vi "REF_X_COM8_hex_VE_FP_STOP_BR_slew_LIM2_Si3540.vi"() -> ()   [LabVIEW 2009]
uses:
  <vilib>/Instr/_visa.llb/VISA Configure Serial Port (Instr).vi
panel:
  out "slew velocity mm/sec":dbl
  out "slew length mm":dbl
  in  "Slew Cancel":bool
  out "Position mm":dbl
  out "offset":dbl
  out "mm/rev":dbl
  out "step/rev":u32
  out "rev/sec":dbl
  in  "Slew Length":i32 min=-99000 max=101000 step=100
  out "Slew Ready":bool
  in  "Slew Set":bool
  in  "Slew Go":bool
  in  "Velocity":dbl
  in  "Slew Velocity":dbl=0.0043 min=0.0042 max=0.105 step=0.0042
  in  "Backlash":i32
  in  "Stop":bool
  out "In Range?":bool
  out "Current Values":i32 max=2000
  out "Status":string
  in  "Go":bool
  in  "Move to":i32=-20000 min=-100000 max=100000 step=500
  out "MINPOS":i32=-94296
  out "MAXPOS":i32=-34296
  out "COM PORT":refnum<visa-resource-name>="COM5"
  # "REF Y"
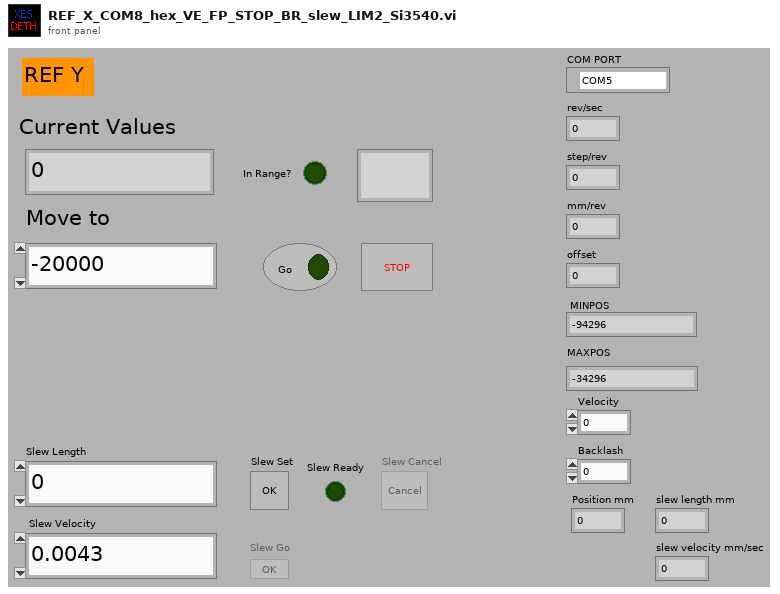
[diagram p1: front panel]
types:
  T1 = enum8{"Enabled", "Disabled", "Disabled and Grayed Out"}
  T2 = enum16{"Power-up Signature", "Accel Rate", "Accel Max", "Bit Rate", "Buffer Status", "Change Current", "Commence Jogging", "Change Jog Speed", "Continue", "Define Address", "Distance for FC,FM,FO,FY", "Decel Rate", "Distance or Position", "Define Limits", "Encoder Deadband", "Encoder Function", "Encoder Position", "Encoder Ratio", "Feed to Length with Speed Change", "Feed to Length", "Feed to Sensor with Mask Dist", "Feed to Length & Set Output", "Feed to Position", "Feed to Sensor", "Feed to Sensor w/safety", "Follow Handwheel", "Immediate Distance?", "Immediate Encoder?", "Immediate Low Output", "Immediate High Output", "Immediate Position?", "Input Status?", "Jog Accel/Decel", "Jog Disable", "Jog Enable", "Jog Speed", "Motor Disable", "Motor Enable", "Microstep Resolution", "Power up Current", "Power up Mode", "Pause", "Request Status", "Revision Level?", "Seek Home", "Stop Jogging", "Stop & Kill Buffer", "Set Output", "Set ABS Position", "Send String", "Stop", "Velocity for Speed Change", "Velocity Setting", "Wait for Input", "Wait Time"}
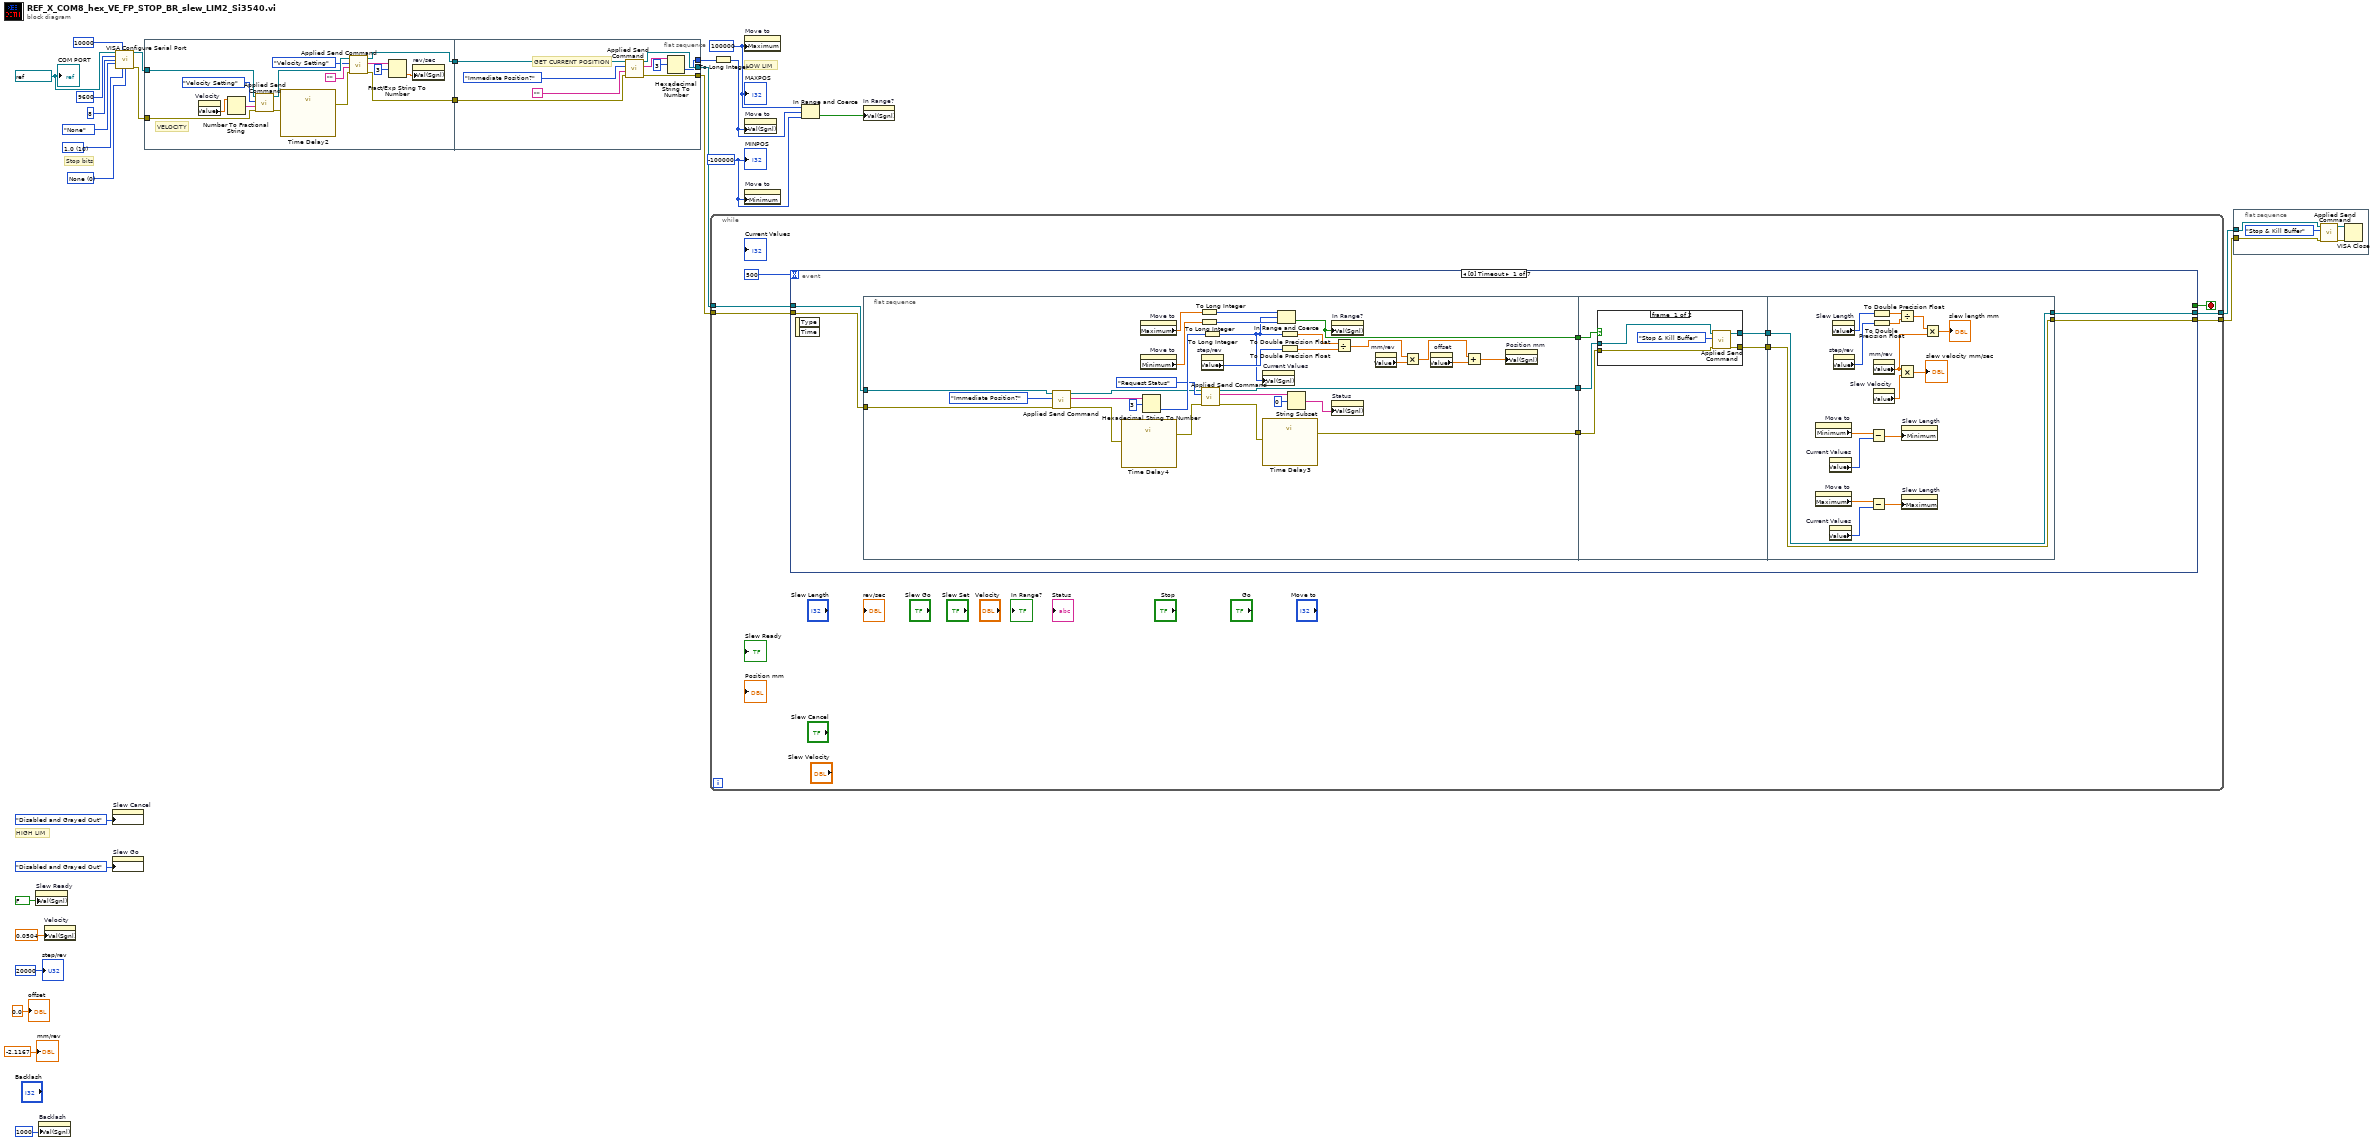
[diagram p0: block diagram]
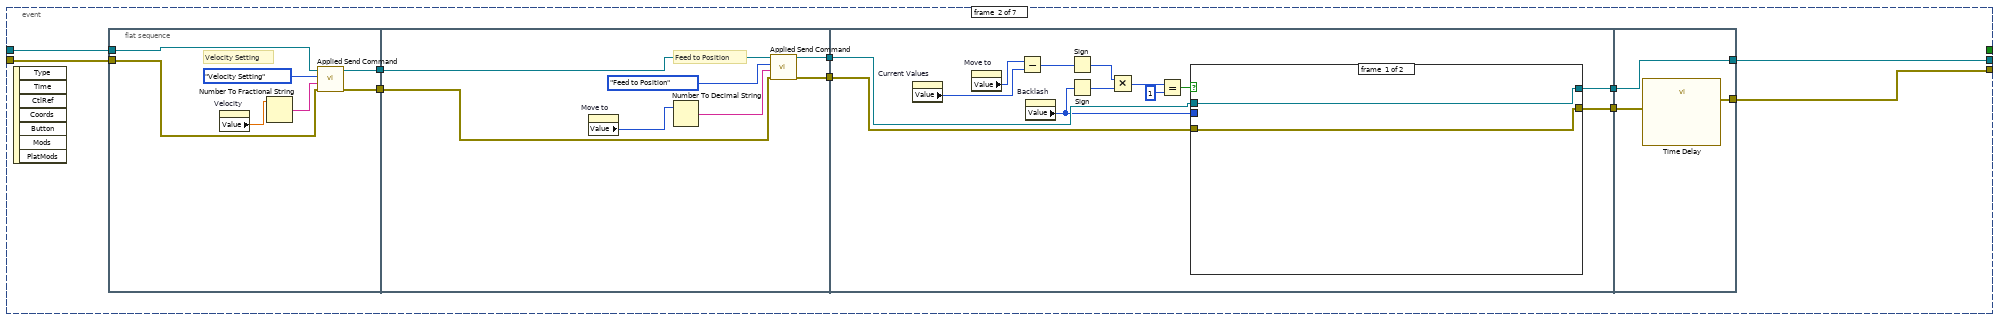
[diagram p3: hidden frame]
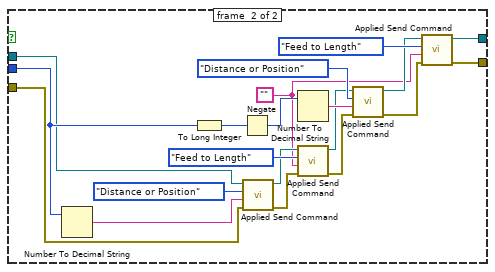
[diagram p4: hidden frame]
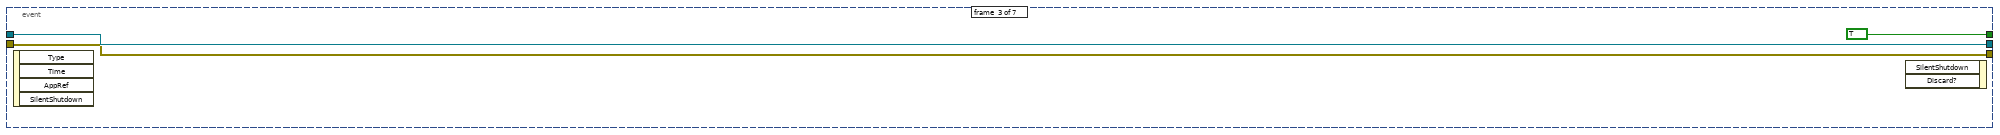
[diagram p5: hidden frame]
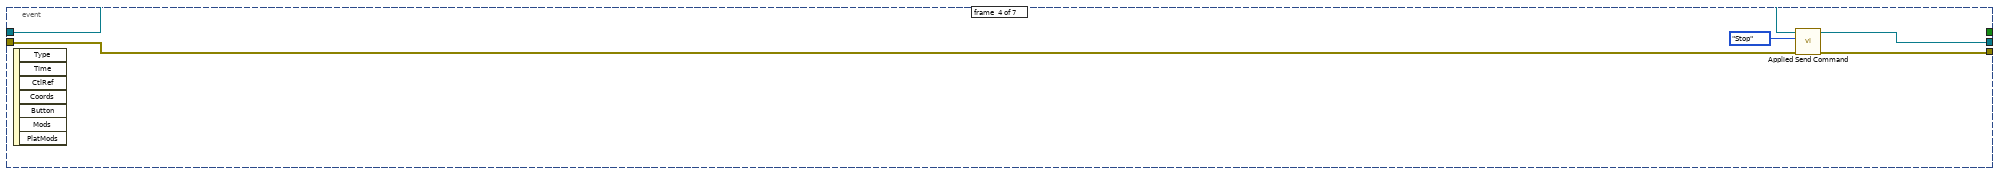
[diagram p6: hidden frame]
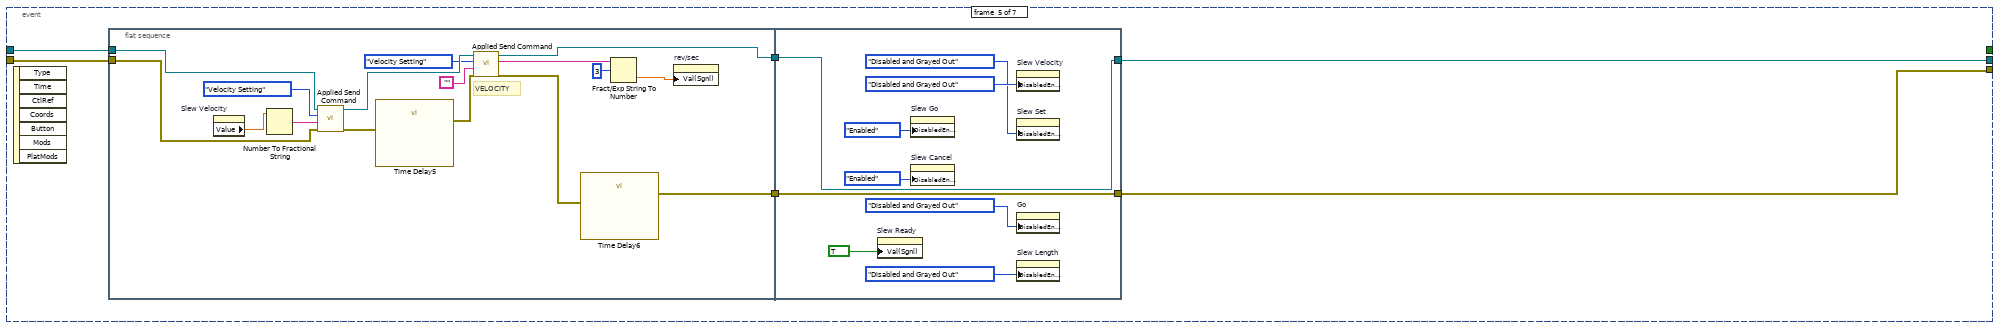
[diagram p7: hidden frame]
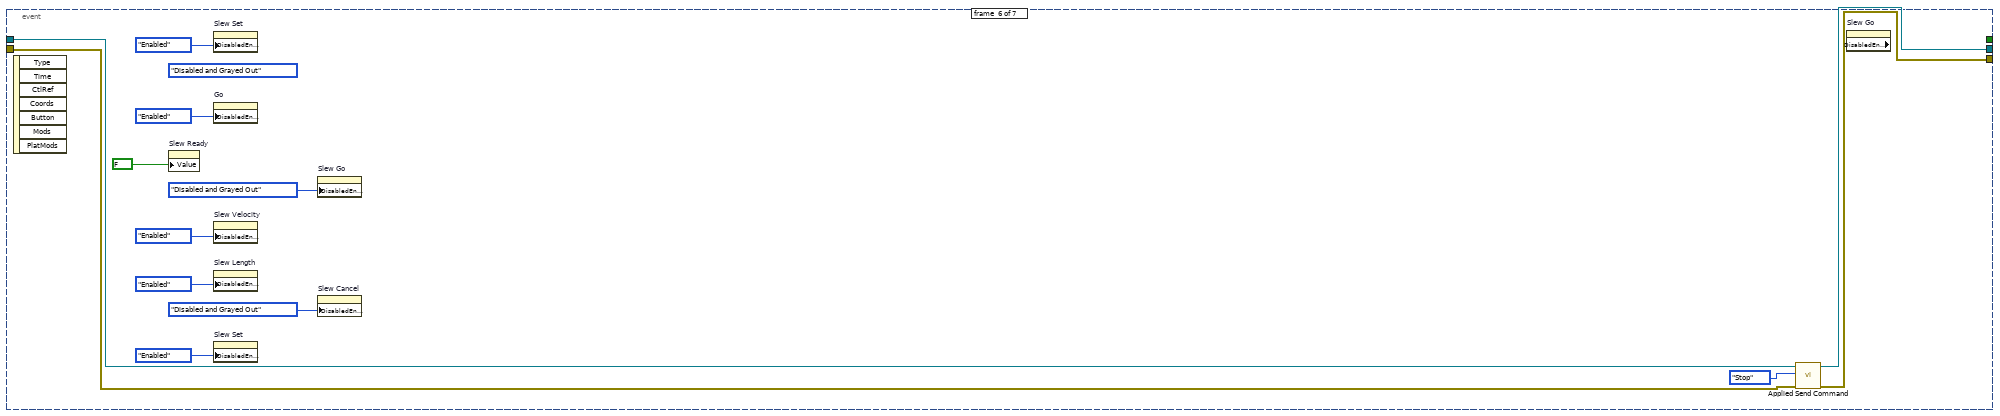
[diagram p8: hidden frame]
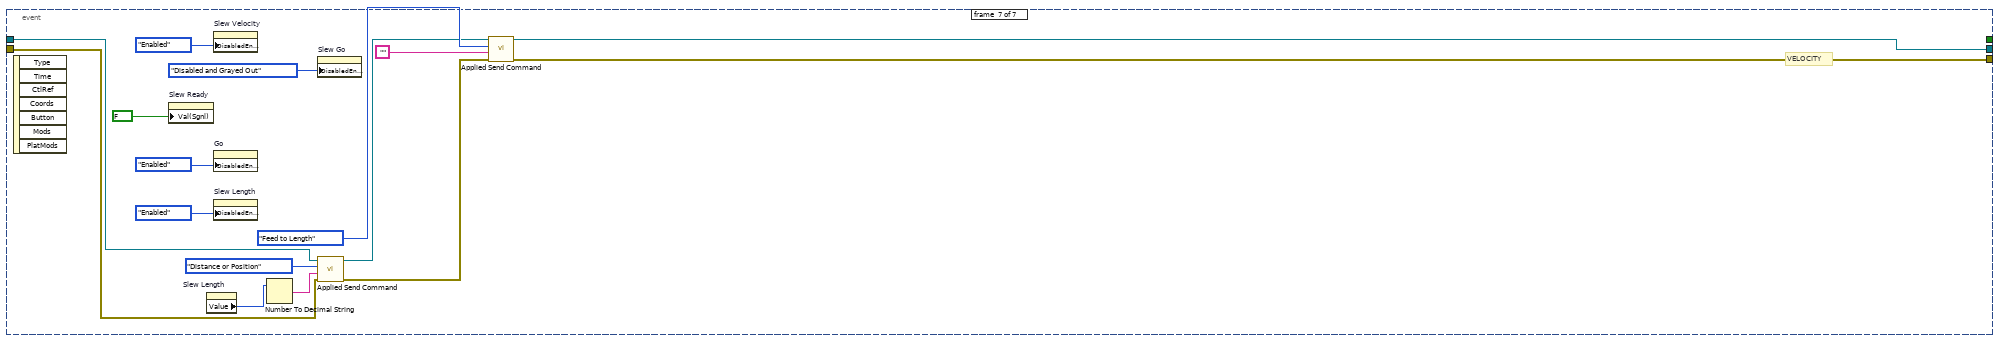
[diagram p9: hidden frame]
diagram:
  w14 = -100000 ("lower limit")
  w13 = 100000 ("upper limit")
  w22 = refnum<visa-resource-name> "COM8" ("COM PORT")
  w24 = u16 0 items=["None", "XON/XOFF", "RTS/CTS", "XON/XOFF & RTS/CTS", "DTR/DSR", "XON/XOFF & DTR/DSR"] ("flow control (0:none)")
  w25 = u16 10 items=["1.0"=10, "1.5"=15, "2.0"=20] ("stop bits (10: 1 bit)")
  # "HIGH LIM"
  # "LOW LIM"
  # "Stop bits"
  n1 = property on="Slew Ready" class="Bool (strict)"("Val(Sgnl)"=FALSE ("Value (Signaling)")) -> ()  [unwired: 2 in, 2 out]
  n2 = property on="Backlash" class="DigNum (strict)"("Val(Sgnl)"=u32 1000 ("Value (Signaling)")) -> ()  [unwired: 2 in, 2 out]
  n3 = property on="Velocity" class="DigNum (strict)"("Val(Sgnl)"=0.0504 ("Value (Signaling)")) -> ()  [unwired: 2 in, 2 out]
  n4 = property on="Slew Cancel" class="Bool"("DisabledEnum"=T1."Disabled and Grayed Out" ("Disabled")) -> ()  [unwired: 2 in, 2 out]
  n5 = property on="Slew Go" class="Bool"("DisabledEnum"=T1."Disabled and Grayed Out" ("Disabled")) -> ()  [unwired: 2 in, 2 out]
  n6 = call-poly "VISA Configure Serial Port"("VISA resource name"=w22, "timeout (10sec)"=u32 10000, "baud rate (9600)"=u32 9600, "data bits (8)"=u16 8, "parity (0:none)"=enum16{"None", "Odd", "Even", "Mark", "Space"}."None", "stop bits (10: 1 bit)"=w25, "flow control (0:none)"=w24) -> ("VISA resource name out"=w8:refnum<visa-resource-name>, "error out"=w7:errorcluster)  [unwired: 7 in]
  n7 = flat-sequence {
    tunnel: [w35] -> w10
    tunnel: [w36] -> w9
    tunnel: w8 -> [w34]
    tunnel: w7 -> [w33]
    tunnel: [w52] -> w21
    tunnel: [w51] -> w20
    tunnel: [w44] -> w11
    tunnel: w10 -> [w50]
    tunnel: w9 -> [w49]
    frame #0 {
      # "VELOCITY"
      n8 = property on="Velocity" class="DigNum (strict)"() -> ("Value"=w31:dbl)  [unwired: 2 in, 2 out]
      n9 = Number To Fractional String(number=w31) -> (F-format string=w30:string)  [unwired: 3 in]
      n10 = call "Applied Send Command.vi"("error in (no error)"=w33, "Extra"=w30, "Command"=T2."Velocity Setting", "VISA resource name"=w34) -> ("error out"=w32:errorcluster, "VISA resource name out"=w43:refnum<visa-resource-name>)  [unwired: 3 in, 1 out]
      n11 = call "Time Delay2"("error in (no error)"=w32) -> ("error out"=w41:errorcluster)  [unwired: 10 in]
      n12 = call "Applied Send Command.vi"("error in (no error)"=w41, "Extra"="", "Command"=T2."Velocity Setting", "VISA resource name"=w43) -> ("error out"=w36:errorcluster, "read buffer"=w39:string, "VISA resource name out"=w35:refnum<visa-resource-name>)  [unwired: 3 in]
      n13 = Fract/Exp String To Number(string=w39, offset=3) -> (number=w29:dbl)  [unwired: 2 in, 1 out]
      n14 = property on="rev/sec" class="DigNum (strict)"("Val(Sgnl)"=w29) -> ()  [unwired: 2 in, 2 out]
    }
    frame #1 {
      # "GET CURRENT POSITION"
      n15 = call "Applied Send Command.vi"("error in (no error)"=w49, "Extra"="", "Command"=T2."Immediate Position?", "VISA resource name"=w50) -> ("error out"=w51:errorcluster, "read buffer"=w47:string, "VISA resource name out"=w52:refnum<visa-resource-name>)  [unwired: 3 in]
      n16 = Hexadecimal String To Number(string=w47, offset=3) -> (number=w44:u32)  [unwired: 1 in, 1 out]
    }
  }
  n17 = while {
    tunnel: w21 -> [w54]
    tunnel: w20 -> [w57]
    tunnel: [w58] -> w17
    tunnel: [w56] -> w18
    stop <- w53 stop-if-true
    n18 = event shown="[0] Timeout" {
      selector: _ -> [_ _ _ _ _ _ _]
      dyn-events: _ -> [_ _ _ _ _ _ _]
      timeout: 500 -> [_ _ _ _ _ _ _]
      tunnel: w57 -> [w67 w136 w190 w194 w202 w232 w242]
      tunnel: [w66 w133 w190 w192 w200 w234 w248] -> w58
      tunnel: w54 -> [w64 w135 w191 w195 w201 w233 w244]
      tunnel: [w65 w134 w191 w193 w197 w235 w249] -> w56
      tunnel: [_ _ TRUE _ _ _ _] -> w53
      event #0 {
        n19 = event-data() -> ()  [unwired: 1 in, 2 out]
        n20 = flat-sequence {
          tunnel: w67 -> [w88]
          tunnel: w64 -> [w87]
          tunnel: [w97] -> w63
          tunnel: [w89] -> w61
          tunnel: [w77] -> w59
          tunnel: w63 -> [w99]
          tunnel: [w100] -> w62
          tunnel: w61 -> [w102]
          tunnel: [w101] -> w60
          tunnel: w59 -> [w98]
          tunnel: [w125] -> w66
          tunnel: [w126] -> w65
          tunnel: w62 -> [w126]
          tunnel: w60 -> [w125]
          frame #0 {
            n21 = call "Applied Send Command.vi"("error in (no error)"=w88, "Command"=T2."Immediate Position?", "VISA resource name"=w87) -> ("error out"=w84:errorcluster, "read buffer"=w95:string, "VISA resource name out"=w91:refnum<visa-resource-name>)  [unwired: 4 in]
            n22 = call "Time Delay4"("error in (no error)"=w84) -> ("error out"=w83:errorcluster)  [unwired: 10 in]
            n23 = property on="Move to" class="DigNum (strict)"() -> ("Maximum"=w79:dbl)  [unwired: 2 in, 2 out]
            n24 = property on="Move to" class="DigNum (strict)"() -> ("Minimum"=w81:dbl)  [unwired: 2 in, 2 out]
            n25 = Hexadecimal String To Number(string=w95, offset=3) -> (number=w94:u32)  [unwired: 1 in, 1 out]
            n26 = To Long Integer(number=w79) -> (32bit integer=w78:i32)
            n27 = To Long Integer(number=w81) -> (32bit integer=w80:i32)
            n28 = call "Applied Send Command.vi"("error in (no error)"=w83, "Command"=T2."Request Status", "VISA resource name"=w91) -> ("error out"=w90:errorcluster, "read buffer"=w86:string, "VISA resource name out"=w97:refnum<visa-resource-name>)  [unwired: 4 in]
            n29 = property on="step/rev" class="DigNum (strict)"() -> ("Value"=w75:u32)  [unwired: 2 in, 2 out]
            n30 = To Long Integer(number=w94) -> (32bit integer=w69:i32)
            n31 = property on="Current Values" class="DigNum (strict)"("Val(Sgnl)"=w69) -> ()  [unwired: 2 in, 2 out]
            n32 = call "Time Delay3"("error in (no error)"=w90) -> ("error out"=w89:errorcluster)  [unwired: 10 in]
            n33 = In Range and Coerce(upper limit=w78, x=w69, lower limit=w80) -> (In Range?=w77:bool)  [unwired: 1 out]
            n34 = To Double Precision Float(number=w69) -> (double precision float=w70:dbl)
            n35 = To Double Precision Float(number=w75) -> (double precision float=w76:dbl)
            n36 = String Subset(string=w86, offset (0)=0) -> (substring=w82:string)  [unwired: 1 in]
            n37 = property on="In Range?" class="Bool (strict)"("Val(Sgnl)"=w77) -> ()  [unwired: 2 in, 2 out]
            n38 = property on="Status" class="Str"("Val(Sgnl)"=w82) -> ()  [unwired: 2 in, 2 out]
            n39 = Divide(x=w70, y=w76) -> (x/y=w74:dbl)
            n40 = property on="mm/rev" class="DigNum (strict)"() -> ("Value"=w73:dbl)  [unwired: 2 in, 2 out]
            n41 = Multiply(x=w74, y=w73) -> (x*y=w72:dbl)
            n42 = property on="offset" class="DigNum (strict)"() -> ("Value"=w71:dbl)  [unwired: 2 in, 2 out]
            n43 = Add(x=w72, y=w71) -> (x+y=w68:dbl)
            n44 = property on="Position mm" class="DigNum (strict)"("Val(Sgnl)"=w68) -> ()  [unwired: 2 in, 2 out]
          }
          frame #1 {
            n45 = case shown="False" w98 {
              tunnel: w99 -> [w104 w109]
              tunnel: [w106 w109] -> w100
              tunnel: [w107 w108] -> w101
              tunnel: w102 -> [w103 w108]
              frame #0 {
                n46 = call "Applied Send Command.vi"("error in (no error)"=w103, "Command"=T2."Stop & Kill Buffer", "VISA resource name"=w104) -> ("error out"=w107:errorcluster, "VISA resource name out"=w106:refnum<visa-resource-name>)  [unwired: 4 in, 1 out]
              }
              frame #1 {
              }
            }
          }
          frame #2 {
            n47 = property on="Move to" class="DigNum (strict)"() -> ("Minimum"=w122:dbl)  [unwired: 2 in, 2 out]
            n48 = property on="Move to" class="DigNum (strict)"() -> ("Maximum"=w120:dbl)  [unwired: 2 in, 2 out]
            n49 = property on="Current Values" class="DigNum (strict)"() -> ("Value"=w124:i32)  [unwired: 2 in, 2 out]
            n50 = property on="Current Values" class="DigNum (strict)"() -> ("Value"=w121:i32)  [unwired: 2 in, 2 out]
            n51 = property on="Slew Length" class="DigNum (strict)"() -> ("Value"=w116:i32)  [unwired: 2 in, 2 out]
            n52 = property on="step/rev" class="DigNum (strict)"() -> ("Value"=w114:u32)  [unwired: 2 in, 2 out]
            n53 = Subtract(x=w122, y=w124) -> (x-y=w123:dbl)
            n54 = Subtract(x=w120, y=w121) -> (x-y=w119:dbl)
            n55 = To Double Precision Float(number=w116) -> (double precision float=w115:dbl)
            n56 = To Double Precision Float(number=w114) -> (double precision float=w118:dbl)
            n57 = property on="mm/rev" class="DigNum (strict)"() -> ("Value"=w110:dbl)  [unwired: 2 in, 2 out]
            n58 = property on="Slew Velocity" class="DigNum (strict)"() -> ("Value"=w112:dbl)  [unwired: 2 in, 2 out]
            n59 = Divide(x=w115, y=w118) -> (x/y=w117:dbl)
            n60 = Multiply(x=w110, y=w112) -> (x*y=→"slew velocity mm/sec":dbl)
            n61 = property on="Slew Length" class="DigNum (strict)"("Minimum"=w123) -> ()  [unwired: 2 in, 2 out]
            n62 = property on="Slew Length" class="DigNum (strict)"("Maximum"=w119) -> ()  [unwired: 2 in, 2 out]
            n63 = Multiply(x=w117, y=w110) -> (x*y=→"slew length mm":dbl)
          }
        }
      }
      event #1 {
        n64 = event-data() -> ()  [unwired: 1 in, 7 out]
        n65 = flat-sequence {
          tunnel: w135 -> [w139]
          tunnel: w136 -> [w142]
          tunnel: [w141] -> w129
          tunnel: [w140] -> w128
          tunnel: w129 -> [w149]
          tunnel: w128 -> [w150]
          tunnel: [w147] -> w132
          tunnel: [w146] -> w130
          tunnel: w132 -> [w163]
          tunnel: [w160] -> w131
          tunnel: w130 -> [w162]
          tunnel: [w161] -> w127
          tunnel: [w187] -> w133
          tunnel: [w188] -> w134
          tunnel: w131 -> [w188]
          tunnel: w127 -> [w186]
          frame #0 {
            # "Velocity Setting"
            n66 = property on="Velocity" class="DigNum (strict)"() -> ("Value"=w143:dbl)  [unwired: 2 in, 2 out]
            n67 = Number To Fractional String(number=w143) -> (F-format string=w138:string)  [unwired: 3 in]
            n68 = call "Applied Send Command.vi"("error in (no error)"=w142, "Extra"=w138, "Command"=T2."Velocity Setting", "VISA resource name"=w139) -> ("error out"=w141:errorcluster, "VISA resource name out"=w140:refnum<visa-resource-name>)  [unwired: 3 in, 1 out]
          }
          frame #1 {
            # "Feed to Position"
            n69 = property on="Move to" class="DigNum (strict)"() -> ("Value"=w145:i32)  [unwired: 2 in, 2 out]
            n70 = Number To Decimal String(number=w145) -> (decimal integer string=w144:string)  [unwired: 1 in]
            n71 = call "Applied Send Command.vi"("error in (no error)"=w149, "Extra"=w144, "Command"=T2."Feed to Position", "VISA resource name"=w150) -> ("error out"=w146:errorcluster, "VISA resource name out"=w147:refnum<visa-resource-name>)  [unwired: 3 in, 1 out]
          }
          frame #2 {
            n72 = property on="Current Values" class="DigNum (strict)"() -> ("Value"=w158:i32)  [unwired: 2 in, 2 out]
            n73 = property on="Move to" class="DigNum (strict)"() -> ("Value"=w159:i32)  [unwired: 2 in, 2 out]
            n74 = Subtract(x=w159, y=w158) -> (x-y=w157:i32)
            n75 = property on="Backlash" class="DigNum (strict)"() -> ("Value"=w151:i32)  [unwired: 2 in, 2 out]
            n76 = Sign(1:w157) -> (0:w156:i32)
            n77 = Sign(1:w151) -> (0:w155:i32)
            n78 = Multiply(x=w156, y=w155) -> (x*y=w154:i32)
            n79 = Equal?(x=w154, y=1) -> (x = y?=w152:bool)
            n80 = case shown="True" w152 {
              tunnel: w163 -> [w165 w177]
              tunnel: [w165 w183] -> w160
              tunnel: [w164 w184] -> w161
              tunnel: w162 -> [w164 w176]
              tunnel: w151 -> [_ w179]
              frame #0 {
              }
              frame #1 {
                w166 = ""
                n81 = Number To Decimal String(number=w179) -> (decimal integer string=w172:string)  [unwired: 1 in]
                n82 = To Long Integer(number=w179) -> (32bit integer=w181:i32)
                n83 = Negate(x=w181) -> (-x=w182:i32)
                n84 = call "Applied Send Command.vi"("error in (no error)"=w176, "Extra"=w172, "Command"=T2."Distance or Position", "VISA resource name"=w177) -> ("error out"=w173:errorcluster, "VISA resource name out"=w174:refnum<visa-resource-name>)  [unwired: 3 in, 1 out]
                n85 = Number To Decimal String(number=w182) -> (decimal integer string=w171:string)  [unwired: 1 in]
                n86 = call "Applied Send Command.vi"("error in (no error)"=w173, "Extra"=w166, "Command"=T2."Feed to Length", "VISA resource name"=w174) -> ("error out"=w169:errorcluster, "VISA resource name out"=w170:refnum<visa-resource-name>)  [unwired: 3 in, 1 out]
                n87 = call "Applied Send Command.vi"("error in (no error)"=w169, "Extra"=w171, "Command"=T2."Distance or Position", "VISA resource name"=w170) -> ("error out"=w167:errorcluster, "VISA resource name out"=w168:refnum<visa-resource-name>)  [unwired: 3 in, 1 out]
                n88 = call "Applied Send Command.vi"("error in (no error)"=w167, "Extra"=w166, "Command"=T2."Feed to Length", "VISA resource name"=w168) -> ("error out"=w184:errorcluster, "VISA resource name out"=w183:refnum<visa-resource-name>)  [unwired: 3 in, 1 out]
              }
            }
          }
          frame #3 {
            n89 = call "Time Delay"("error in (no error)"=w186) -> ("error out"=w187:errorcluster)  [unwired: 10 in]
          }
        }
      }
      event #2 {
        n90 = event-data() -> ()  [unwired: 1 in, 4 out]
        n91 = event-data() -> ()  [unwired: 3 in, 1 out]
      }
      event #3 {
        n92 = event-data() -> ()  [unwired: 1 in, 7 out]
        n93 = call "Applied Send Command.vi"("error in (no error)"=w194, "Command"=T2."Stop", "VISA resource name"=w195) -> ("error out"=w192:errorcluster, "VISA resource name out"=w193:refnum<visa-resource-name>)  [unwired: 4 in, 1 out]
      }
      event #4 {
        n94 = event-data() -> ()  [unwired: 1 in, 7 out]
        n95 = flat-sequence {
          tunnel: w202 -> [w209]
          tunnel: w201 -> [w208]
          tunnel: [w205] -> w199
          tunnel: [w203] -> w198
          tunnel: [w226] -> w200
          tunnel: [w227] -> w197
          tunnel: w199 -> [w227]
          tunnel: w198 -> [w226]
          frame #0 {
            # "VELOCITY"
            n96 = property on="Slew Velocity" class="DigNum (strict)"() -> ("Value"=w206:dbl)  [unwired: 2 in, 2 out]
            n97 = Number To Fractional String(number=w206) -> (F-format string=w207:string)  [unwired: 3 in]
            n98 = call "Applied Send Command.vi"("error in (no error)"=w209, "Extra"=w207, "Command"=T2."Velocity Setting", "VISA resource name"=w208) -> ("error out"=w210:errorcluster, "VISA resource name out"=w218:refnum<visa-resource-name>)  [unwired: 3 in, 1 out]
            n99 = call "Time Delay5"("error in (no error)"=w210) -> ("error out"=w215:errorcluster)  [unwired: 10 in]
            n100 = call "Applied Send Command.vi"("error in (no error)"=w215, "Extra"="", "Command"=T2."Velocity Setting", "VISA resource name"=w218) -> ("error out"=w204:errorcluster, "read buffer"=w213:string, "VISA resource name out"=w205:refnum<visa-resource-name>)  [unwired: 3 in]
            n101 = call "Time Delay6"("error in (no error)"=w204) -> ("error out"=w203:errorcluster)  [unwired: 10 in]
            n102 = Fract/Exp String To Number(string=w213, offset=3) -> (number=w217:dbl)  [unwired: 2 in, 1 out]
            n103 = property on="rev/sec" class="DigNum (strict)"("Val(Sgnl)"=w217) -> ()  [unwired: 2 in, 2 out]
          }
          frame #1 {
            n104 = property on="Slew Ready" class="Bool (strict)"("Val(Sgnl)"=TRUE ("Slew Ready 2")) -> ()  [unwired: 2 in, 2 out]
            n105 = property on="Slew Go" class="Bool"("DisabledEnum"=T1."Enabled" ("Disabled")) -> ()  [unwired: 2 in, 2 out]
            n106 = property on="Slew Cancel" class="Bool"("DisabledEnum"=T1."Enabled" ("Disabled")) -> ()  [unwired: 2 in, 2 out]
            n107 = property on="Slew Velocity" class="DigNum (strict)"("DisabledEnum"=T1."Disabled and Grayed Out" ("Disabled")) -> ()  [unwired: 2 in, 2 out]
            n108 = property on="Slew Set" class="Bool"("DisabledEnum"=T1."Disabled and Grayed Out" ("Disabled")) -> ()  [unwired: 2 in, 2 out]
            n109 = property on="Go" class="Bool"("DisabledEnum"=T1."Disabled and Grayed Out" ("Disabled")) -> ()  [unwired: 2 in, 2 out]
            n110 = property on="Slew Length" class="DigNum (strict)"("DisabledEnum"=T1."Disabled and Grayed Out" ("Disabled")) -> ()  [unwired: 2 in, 2 out]
          }
        }
      }
      event #5 {
        (unwired) T1."Disabled and Grayed Out" ("Disabled")
        n111 = event-data() -> ()  [unwired: 1 in, 7 out]
        n112 = property on="Slew Ready" class="Bool (strict)"("Value"=FALSE ("Slew Ready")) -> ()  [unwired: 2 in, 2 out]
        n113 = property on="Slew Set" class="Bool"("DisabledEnum"=T1."Enabled" ("Disabled")) -> ()  [unwired: 2 in, 2 out]
        n114 = property on="Go" class="Bool"("DisabledEnum"=T1."Enabled" ("Disabled")) -> ()  [unwired: 2 in, 2 out]
        n115 = property on="Slew Velocity" class="DigNum (strict)"("DisabledEnum"=T1."Enabled" ("Disabled")) -> ()  [unwired: 2 in, 2 out]
        n116 = property on="Slew Length" class="DigNum (strict)"("DisabledEnum"=T1."Enabled" ("Disabled")) -> ()  [unwired: 2 in, 2 out]
        n117 = property on="Slew Set" class="Bool"("DisabledEnum"=T1."Enabled" ("Disabled")) -> ()  [unwired: 2 in, 2 out]
        n118 = property on="Slew Go" class="Bool"("DisabledEnum"=T1."Disabled and Grayed Out" ("Disabled")) -> ()  [unwired: 2 in, 2 out]
        n119 = property on="Slew Cancel" class="Bool"("DisabledEnum"=T1."Disabled and Grayed Out" ("Disabled")) -> ()  [unwired: 2 in, 2 out]
        n120 = call "Applied Send Command.vi"("error in (no error)"=w232, "Command"=T2."Stop", "VISA resource name"=w233) -> ("error out"=w234:errorcluster, "VISA resource name out"=w235:refnum<visa-resource-name>)  [unwired: 4 in, 1 out]
        n121 = property on="Slew Go" class="Bool" props=["DisabledEnum"]() -> ()  [unwired: 2 in, 3 out]
      }
      event #6 {
        # "VELOCITY"
        n122 = event-data() -> ()  [unwired: 1 in, 7 out]
        n123 = property on="Slew Ready" class="Bool (strict)"("Val(Sgnl)"=FALSE ("Slew Ready 2")) -> ()  [unwired: 2 in, 2 out]
        n124 = property on="Slew Length" class="DigNum (strict)"() -> ("Value"=w250:i32)  [unwired: 2 in, 2 out]
        n125 = property on="Slew Velocity" class="DigNum (strict)"("DisabledEnum"=T1."Enabled" ("Disabled")) -> ()  [unwired: 2 in, 2 out]
        n126 = property on="Go" class="Bool"("DisabledEnum"=T1."Enabled" ("Disabled")) -> ()  [unwired: 2 in, 2 out]
        n127 = property on="Slew Length" class="DigNum (strict)"("DisabledEnum"=T1."Enabled" ("Disabled")) -> ()  [unwired: 2 in, 2 out]
        n128 = Number To Decimal String(number=w250) -> (decimal integer string=w246:string)  [unwired: 1 in]
        n129 = property on="Slew Go" class="Bool"("DisabledEnum"=T1."Disabled and Grayed Out" ("Disabled")) -> ()  [unwired: 2 in, 2 out]
        n130 = call "Applied Send Command.vi"("error in (no error)"=w242, "Extra"=w246, "Command"=T2."Distance or Position", "VISA resource name"=w244) -> ("error out"=w241:errorcluster, "VISA resource name out"=w243:refnum<visa-resource-name>)  [unwired: 3 in, 1 out]
        n131 = call "Applied Send Command.vi"("error in (no error)"=w241, "Extra"="", "Command"=T2."Feed to Length", "VISA resource name"=w243) -> ("error out"=w248:errorcluster, "VISA resource name out"=w249:refnum<visa-resource-name>)  [unwired: 3 in, 1 out]
      }
    }
  }
  n132 = To Long Integer(number=w11) -> (32bit integer=w19:i32)
  n133 = property on="Move to" class="DigNum (strict)"("Maximum"=w13) -> ()  [unwired: 2 in, 2 out]
  n134 = property on="Move to" class="DigNum (strict)"("Val(Sgnl)"=w19) -> ()  [unwired: 2 in, 2 out]
  n135 = property on="Move to" class="DigNum (strict)"("Minimum"=w14) -> ()  [unwired: 2 in, 2 out]
  n136 = In Range and Coerce(upper limit=w13, x=w19, lower limit=w14) -> (In Range?=w16:bool)  [unwired: 1 out]
  n137 = property on="In Range?" class="Bool (strict)"("Val(Sgnl)"=w16) -> ()  [unwired: 2 in, 2 out]
  n138 = flat-sequence {
    tunnel: w18 -> [w260]
    tunnel: w17 -> [w257]
    frame #0 {
      n139 = call "Applied Send Command.vi"("error in (no error)"=w257, "Command"=T2."Stop & Kill Buffer", "VISA resource name"=w260) -> ("error out"=w258:errorcluster, "VISA resource name out"=w259:refnum<visa-resource-name>)  [unwired: 4 in, 1 out]
      n140 = VISA Close(VISA resource name=w259, error in (no error)=w258) -> ()  [unwired: 1 out]
    }
  }
  "COM PORT" <- w22
  "MINPOS" <- w14
  "MAXPOS" <- w13
  "step/rev" <- u32 20000 ("step/rev")
  "mm/rev" <- -2.1167 ("MM/rev")
  "offset" <- 0.0 ("offset")
